vi "INDIVIDUAL VI's VIA CONTROL.vi"() -> ()   [LabVIEW 2013]
uses:
  <vilib>/myRIO/Instrument Drivers/Onboard IO/DIO/vis/Smart Open.vi
  <vilib>/myRIO/Instrument Drivers/Onboard IO/DIO/vis/Write.vi
  <vilib>/myRIO/Instrument Drivers/Onboard IO/DIO/vis/Open.vi
  <vilib>/myRIO/Common/Instrument Driver Framework/myRIO v1.0/DIO/vis/myRIO v1.1 Open DIO.vi
  <vilib>/myRIO/Common/Instrument Driver Framework/Utilities/vis/Validate Channels.vi
  <vilib>/myRIO/Common/Instrument Driver Framework/myRIO v1.0/DIO/vis/myRIO v1.0 Reserve DIO.vi
  <vilib>/myRIO/Common/Instrument Driver Framework/myRIO v1.0/Resource Manager/vis/myRIO v1.0 Reserve Channel List.vi
  <vilib>/myRIO/Common/Instrument Driver Framework/myRIO v1.0/DIO/vis/myRIO v1.0 Build MUX Configuration DIO.vi
  <vilib>/myRIO/Common/Instrument Driver Framework/myRIO v1.0/Resource Manager/vis/myRIO v1.0 Reserve Channel.vi
  <vilib>/myRIO/Common/Instrument Driver Framework/myRIO v1.0/Resource Manager/vis/myRIO v1.0 Unreserve Channel.vi
  <vilib>/myRIO/Common/Instrument Driver Framework/myRIO v1.0/Resource Manager/vis/myRIO v1.0 Create Configuration List.vi
  <vilib>/myRIO/Common/Instrument Driver Framework/myRIO v1.0/Resource Manager/vis/myRIO v1.0 Build Mutex Name.vi
  <vilib>/myRIO/Common/Instrument Driver Framework/myRIO v1.0/myRIO v1.1 Open.vi
  <vilib>/Utility/VariantDataType/GetNumericInfo.vi
  <vilib>/Utility/error.llb/Error Cluster From Error Code.vi
  <vilib>/myRIO/Common/Instrument Driver Framework/Utilities/vis/IO Manager.vi
  <vilib>/myRIO/Common/Instrument Driver Framework/Utilities/vis/Configuration Manager.vi
  <vilib>/myRIO/Common/Instrument Driver Framework/myRIO v1.0/Resource Manager/vis/myRIO v1.0 Configure IO.vi
  <vilib>/myRIO/Common/Instrument Driver Framework/myRIO v1.0/myRIO v1.0 Close.vi
  <vilib>/myRIO/Common/Instrument Driver Framework/myRIO v1.0/DIO/vis/myRIO v1.0 Write DIO.vi
panel:
  out "Cold Storage":string
  in  "Cold storage":bool
  in  "FERTILIZER":bool
  out "MOISTURE LEVEL(ppm) 2":dbl
  out "HIGH MOISTURE 2":bool
  out "INTERMEDIATE MOISTURE 2":bool=TRUE
  out "LOW MOISTURE 2":bool
  out "CURRENT FARM STATUS":T1(plugin-control)
  in  "WEATHER":bool
  in  "PIC-MAIL-FTP":bool
  in  "DRIVE-SOW":bool
  in  "pH":bool
  in  "SERVO,MOISTURE":bool
  in  "GPS":bool=TRUE
  out "WEATHER FORECAST":T2(array[cluster])
  out "pH VALUE":dbl
  out "LIST OF MOST SUITABLE CROPS":string
  out "POSITION":string="BOT IS IN THE FARM"
  out "Current Longitude [deg]":string="26.882130"
  out "Current Latitude [deg]":string="75.811895"
  out "Alert":bool
  # "SMART AGRICULTURIST SUPPORT SYSTEM"
  # "CONTROLLER"
  # "GPS SECURITY"
  # "REAL TIME MONITORING"
  # "pH SENSOR"
  # "MOISTURE SENSOR"
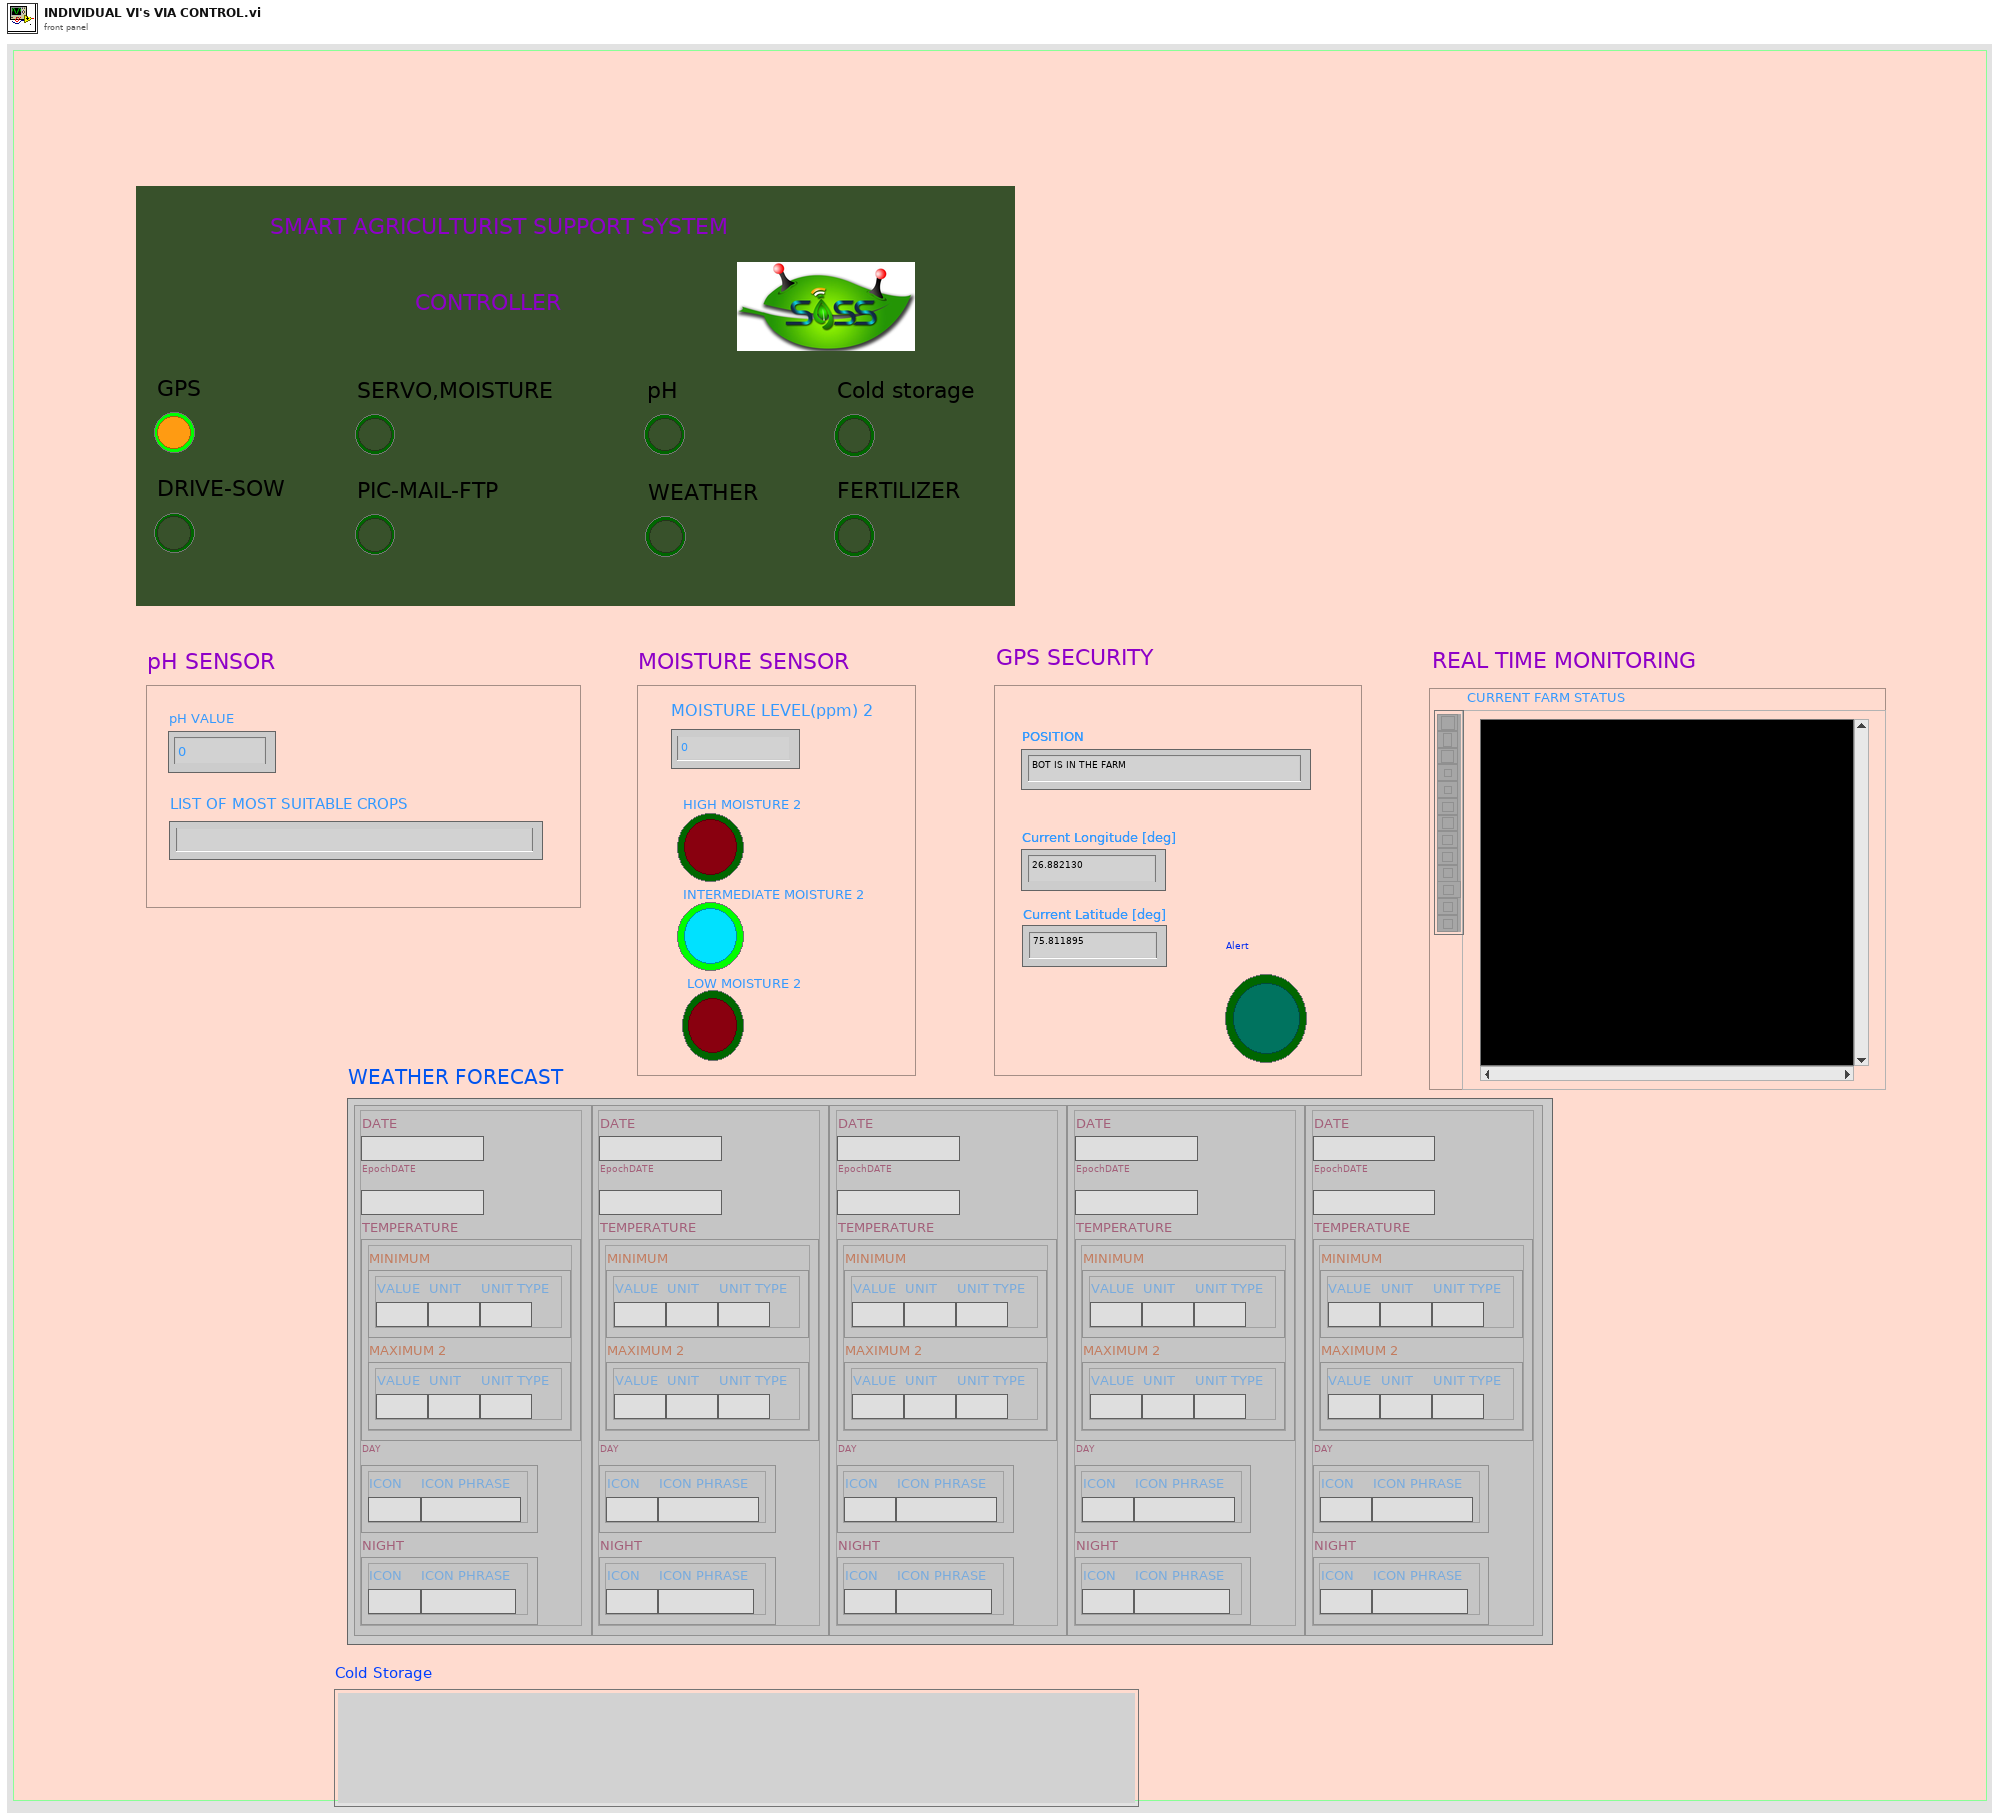
[diagram p1: front panel]
types:
  T1 = typedef "IMAQ Image.ctl" = refnum<image>
  T2 = cluster{"DATE":string, "EpochDATE":string, "TEMPERATURE":cluster{"MINIMUM":cluster{"VALUE":string, "UNIT":string, "UNIT TYPE":string}, "MAXIMUM 2":cluster{"VALUE":string, "UNIT":string, "UNIT TYPE":string}}, "DAY ":cluster{"ICON":string, "ICON PHRASE":string}, "NIGHT":cluster{"ICON":string, "ICON PHRASE":string}}[]
  T3 = cluster{"DATE":string, "EpochDATE":string, "TEMPERATURE":cluster{"MINIMUM":cluster{"VALUE":string, "UNIT":string, "UNIT TYPE 3":string}, "MAXIMUM 2":cluster{"VALUE":string, "UNIT":string, "UNIT TYPE":string}}, "DAY ":cluster{"ICON":string, "ICON PHRASE":string}, "NIGHT":cluster{"ICON":string, "ICON PHRASE":string}}[]
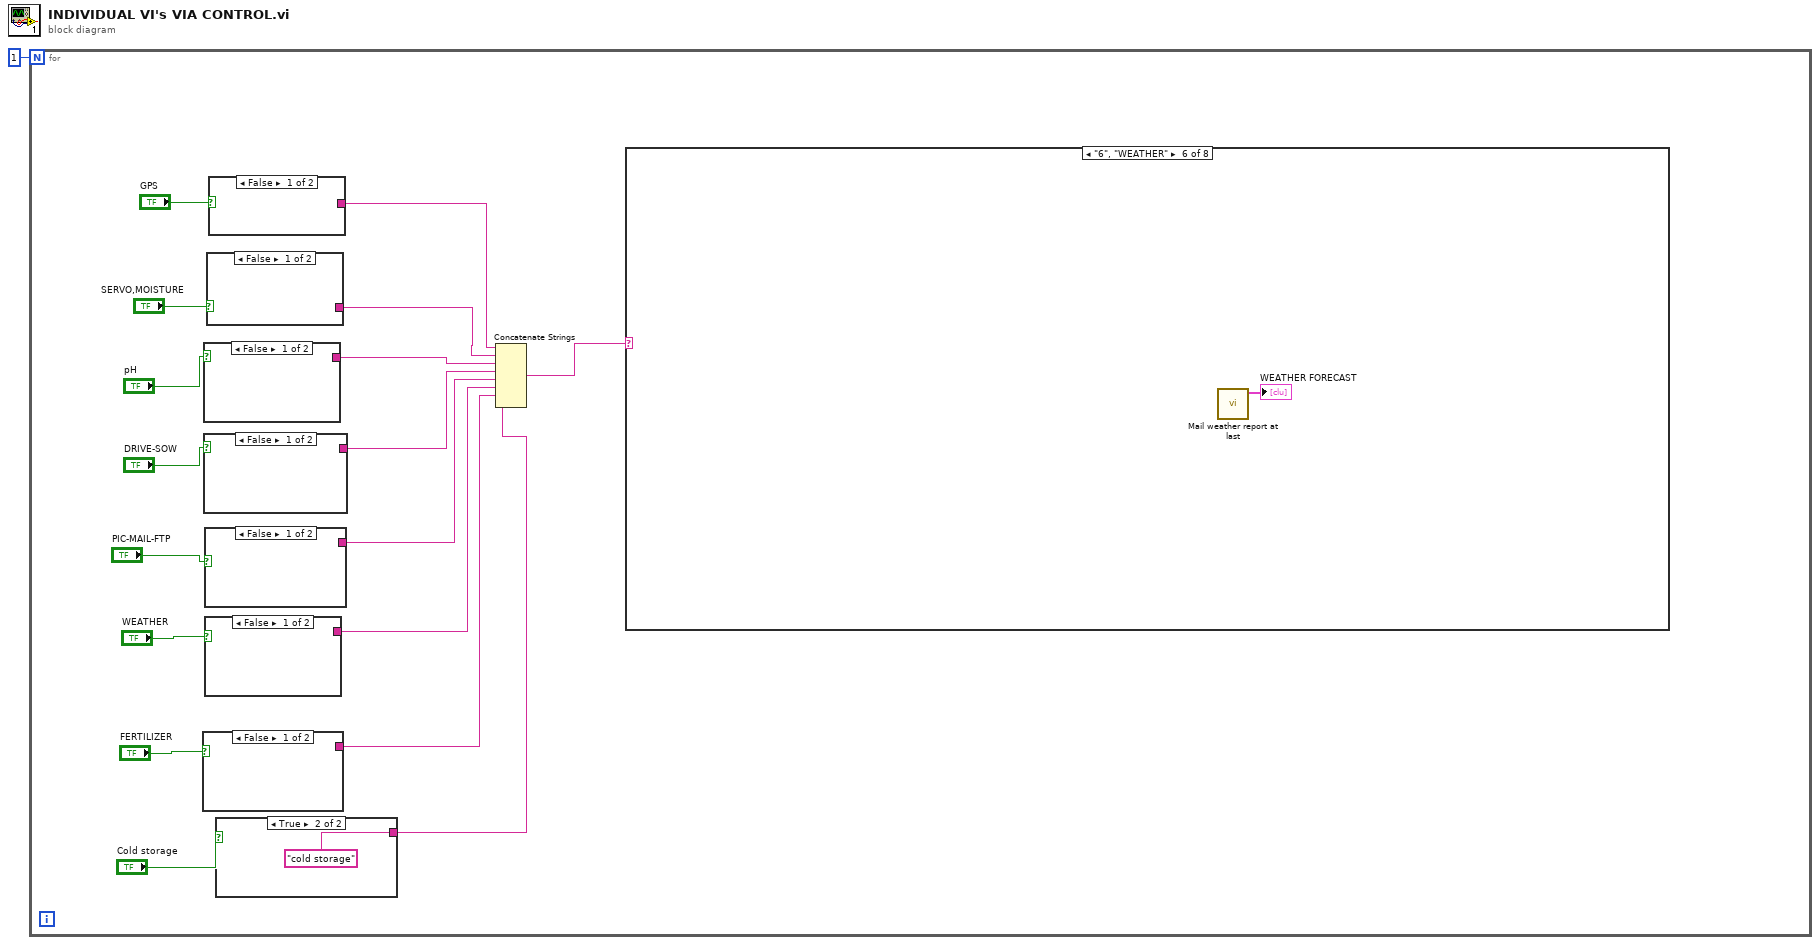
[diagram p0: block diagram]
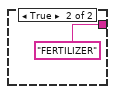
[diagram p3: hidden frame]
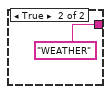
[diagram p4: hidden frame]
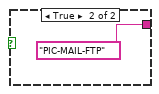
[diagram p5: hidden frame]
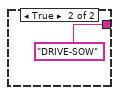
[diagram p6: hidden frame]
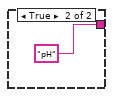
[diagram p7: hidden frame]
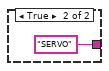
[diagram p8: hidden frame]
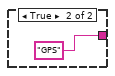
[diagram p9: hidden frame]
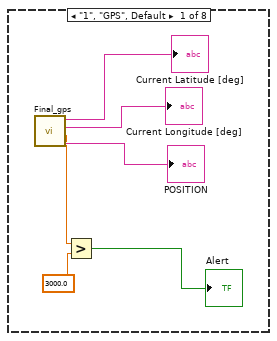
[diagram p10: hidden frame]
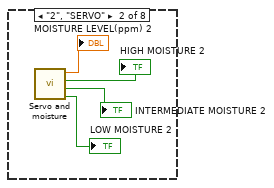
[diagram p11: hidden frame]
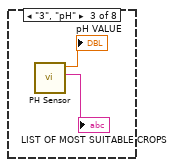
[diagram p12: hidden frame]
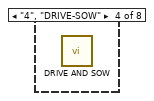
[diagram p13: hidden frame]
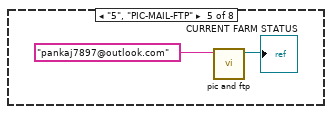
[diagram p14: hidden frame]
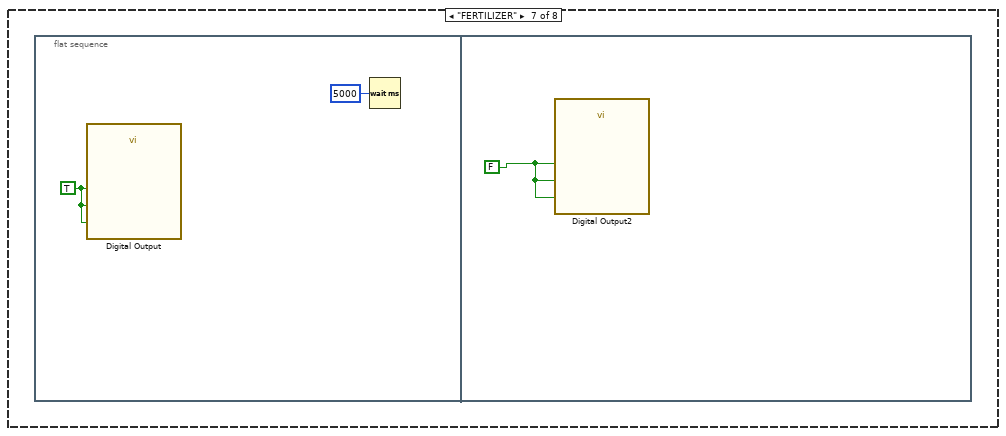
[diagram p15: hidden frame]
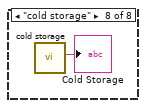
[diagram p16: hidden frame]
diagram:
  n1 = for {
    N: 1 -> [_]
    n2 = case shown="False" "FERTILIZER" {
      tunnel: [_ "FERTILIZER"] -> w4
      frame False {
      }
      frame True {
      }
    }
    n3 = case shown="False" "pH" {
      tunnel: [_ "pH"] -> w11
      frame False {
      }
      frame True {
      }
    }
    n4 = case shown="False" "DRIVE-SOW" {
      tunnel: [_ "DRIVE-SOW"] -> w10
      frame False {
      }
      frame True {
      }
    }
    n5 = case shown="False" "PIC-MAIL-FTP" {
      tunnel: [_ "PIC-MAIL-FTP"] -> w9
      frame False {
      }
      frame True {
      }
    }
    n6 = case shown="False" "WEATHER" {
      tunnel: [_ "WEATHER"] -> w8
      frame False {
      }
      frame True {
      }
    }
    n7 = case shown="False" "SERVO,MOISTURE" {
      tunnel: [_ "SERVO"] -> w7
      frame False {
      }
      frame True {
      }
    }
    n8 = case shown="False" "GPS" {
      tunnel: [_ "GPS"] -> w6
      frame False {
      }
      frame True {
      }
    }
    n9 = case shown="True" "Cold storage" {
      tunnel: [_ "cold storage"] -> w2
      frame False {
      }
      frame True {
      }
    }
    n10 = Concatenate Strings(w6, w7, w11, w10, w9, w8, w4, w2) -> (w17:string)
    n11 = case shown="\"6\", \"WEATHER\"" w17 {
      frame "1", "GPS", Default {
        n12 = call "Final_gps.vi"() -> ("POSITION"=→"POSITION":string, "Distance to Destination m"=w29:dbl, "Current Longitude [deg]"=→"Current Longitude [deg]":string, "Current Latitude [deg]"=→"Current Latitude [deg]":string)  [unwired: 8 in]
        n13 = Greater?(x=w29, y=3000.0) -> (0:→"Alert":bool)
      }
      frame "2", "SERVO" {
        n14 = call "Servo and moisture.vi"() -> ("LOW MOISTURE"=→"LOW MOISTURE 2":bool, "INTERMEDIATE MOISTURE"=→"INTERMEDIATE MOISTURE 2":bool, "HIGH MOISTURE"=→"HIGH MOISTURE 2":bool, "MOISTURE LEVEL(ppm)"=→"MOISTURE LEVEL(ppm) 2":dbl)  [unwired: 8 in]
      }
      frame "3", "pH" {
        n15 = call "PH Sensor.vi"() -> ("SUGGESTED CROP"=→"LIST OF MOST SUITABLE CROPS":string, "pH VALUE"=→"pH VALUE":dbl)  [unwired: 10 in]
      }
      frame "4", "DRIVE-SOW" {
        n16 = call "DRIVE AND SOW.vi"() -> ()  [unwired: 12 in]
      }
      frame "5", "PIC-MAIL-FTP" {
        n17 = call "pic and ftp.vi"("To: 2"="pankaj7897@outlook.com" ("USER EMAIL Id")) -> ("Image Out"=→"CURRENT FARM STATUS":T1)  [unwired: 10 in]
      }
      frame "6", "WEATHER" {
        n18 = call "Mail weather report at last.vi"() -> ("Array 3"=→"WEATHER FORECAST":T3)  [unwired: 11 in]
      }
      frame "FERTILIZER" {
        n19 = flat-sequence {
          frame #0 {
            w43 = TRUE
            n20 = call "Digital Output"("DIR  (A/DIO0 (Pin 11))"=w43, "PWM (A/DIO1 (Pin 13))"=w43, "Fertiliser (A/DIO12 (Pin 22))"=w43) -> ()  [unwired: 24 in, 1 out]
            n21 = Wait (ms)(milliseconds to wait=u32 5000) -> ()  [unwired: 1 out]
          }
          frame #1 {
            w44 = FALSE
            n22 = call "Digital Output2"("DIR (A/DIO0 (Pin 11))"=w44, "PWM (A/DIO1 (Pin 13))"=w44, "Fertiliser (A/DIO12 (Pin 22))"=w44) -> ()  [unwired: 24 in, 1 out]
          }
        }
      }
      frame "cold storage" {
        n23 = call "cold storage.vi"() -> ("Subject 2"=→"Cold Storage":string)  [unwired: 11 in]
      }
    }
  }
